vi "Check Incoming TP Timeouts.vi"(8 "error in":errorcluster, 11 "internal data":T1={"J1939 XNET Settings"={"XNET Database"="", "XNET Cluster"="", "CAN port"="", "Baud rate [Bd]"=0, "J1939 Network Address"=0, "Name"=0, "Termination"=0}, "j1939 queues"={"Processed Outgoing"=refnum, "Process Outgoing"=refnum, "stop notifier"=refnum, "error queue"=refnum, "active dtc"=refnum, "processed inc"=refnum}, "fgv references"={"BAM Buffer"=refnum, "CM Buffer"=refnum, "CM Gen"=refnum, "BAM Gen"=refnum, "Address Claims"=refnum, "RQST"=refnum, "scaling lut"=refnum, "data lut"=refnum, "cyclic scheduler"=refnum}, "frame in"="", "frame out"="", "timing"={"tb to j1939 queue timeout"=100, "j1939 to tb queue timeout"=100, "dtc loop period (ms)"=100, "CAN in loop period (ms)"=100, "process incoming queue timeout (ms)"=100, "Outgoing Write Decimation"=0, "process outgoing loop rate (ms)"=0, "periodic outgoing queue timeout (ms)"=10, "CAN out queue timeout (ms)"=100}}) -> (0 "error out":errorcluster)   [LabVIEW 2013, in "J1939.lvlib"]
uses:
  J1939.lvlib
  API Types/Internal Data.ctl
  API Types/XNET Settings.ctl
  API Types/Setup Information Cluster.ctl
  API Types/CAN Outgoing Message Cluster.ctl
  API Types/Convert DTCs Cluster.ctl
  <vilib>/xnet/xnet.llb/XNET Frame CAN.ctl
  <vilib>/xnet/xnet.llb/XNET Frame Type CAN.ctl
  TP List References.ctl
  BAM/BAM Buffer Connections List_Ref.ctl
  Connection Mode/Connection Mode Generation Connection Ref.ctl
  BAM/BAM Generation Connections List_Ref.ctl
  LUTs/J1939 Address Table Reference.ctl
  RQST/RQST Lookup Table Reference.ctl
  LUTs/J1939 Conversion Lookup Table Reference.ctl
  LUTs/J1939 Data Lookup Table Reference.ctl
  LUTs/Cyclic Frame Scheduler Lut Reference.ctl
  Configuration/TypeDefs/timing configuration.ctl
  TP Connections List State.ctl
  TP Buffer Check Timeout on Connections.vi
  Helpers/Buffer Connections List_Actions.vi
  Common Messages/J1939 Message TP.Conn Abort.vi
  Frame Conversion/Common Conversions.vi
  Frame Conversion/Convert J1939 ID to CAN Arb ID.vi
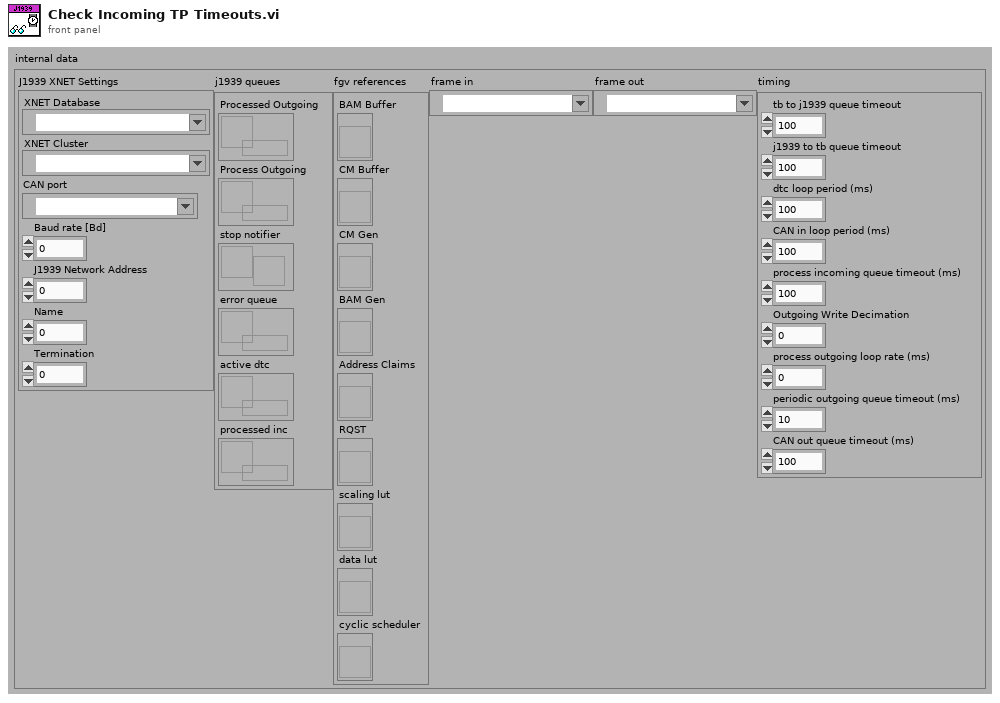
[diagram p1: front panel]
types:
  T1 = typedef "J1939.lvlib/Internal Data.ctl" = cluster{"J1939 XNET Settings":T2, "j1939 queues":T3, "fgv references":T4, "frame in":refnum<k21>, "frame out":refnum<k21>, "timing":T13}
  T2 = typedef "J1939.lvlib/XNET settings.ctl" = cluster{"XNET Database":refnum<k21>, "XNET Cluster":refnum<k21>, "CAN port":refnum<k21>, "Baud rate [Bd]":u32, "J1939 Network Address":u8, "Name":u64, "Termination":u32}
  T3 = typedef "J1939.lvlib/Setup Information Cluster.ctl" = cluster{"Processed Outgoing":refnum<queue>, "Process Outgoing":refnum<queue>, "stop notifier":refnum<notifier>, "error queue":refnum<queue>, "active dtc":refnum<queue>, "processed inc":refnum<queue>}
  T4 = typedef "J1939.lvlib/TP List References.ctl" = cluster{"BAM Buffer":T5, "CM Buffer":T5, "CM Gen":T6, "BAM Gen":T7, "Address Claims":T8, "RQST":T9, "scaling lut":T10, "data lut":T11, "cyclic scheduler":T12}
  T5 = typedef "J1939.lvlib/BAM Buffer Connections List_Ref.ctl" = refnum<vi>
  T6 = typedef "J1939.lvlib/Connection Mode Generation Connection Ref.ctl" = refnum<vi>
  T7 = typedef "J1939.lvlib/BAM Generation Connections List_Ref.ctl" = refnum<vi>
  T8 = typedef "J1939.lvlib/J1939 Address Table Reference.ctl" = refnum<vi>
  T9 = typedef "J1939.lvlib/RQST Lookup Table Reference.ctl" = refnum<vi>
  T10 = typedef "J1939.lvlib/J1939 Conversion Lookup Table Reference.ctl" = refnum<vi>
  T11 = typedef "J1939.lvlib/J1939 Data Lookup Table Reference.ctl" = refnum<vi>
  T12 = typedef "J1939.lvlib/cyclic frame scheduler lut reference.ctl" = refnum<vi>
  T13 = typedef "J1939.lvlib/timing configuration.ctl" = cluster{"tb to j1939 queue timeout":i32, "j1939 to tb queue timeout":i32, "dtc loop period (ms)":i32, "CAN in loop period (ms)":i32, "process incoming queue timeout (ms)":i32, "Outgoing Write Decimation":u32, "process outgoing loop rate (ms)":i32, "periodic outgoing queue timeout (ms)":i32, "CAN out queue timeout (ms)":i32}
  T14 = typedef "J1939.lvlib/TP Connections List State.ctl" = enum16{"Add", "Update", "Get", "Remove", "Initialize"}
  T15 = typedef "J1939.lvlib/TP Buffer Connection Cluster.ctl" = cluster{"Source Address":u8, "Destination Address":u8, "PGN":u32, "Arb ID":u32, "CAN Conversion Index":u32, "Total Expected Bytes":u16, "Total Expected Packets":u8, "Number of Packets Read":u8, "Start Time":u32, "Packets (U8)":u8[], "Timestamp":timestamp}
  T16 = typedef "J1939.lvlib/CAN Outgoing Message Cluster.ctl" = cluster{"Identifier":u32, "Data":u8[]}
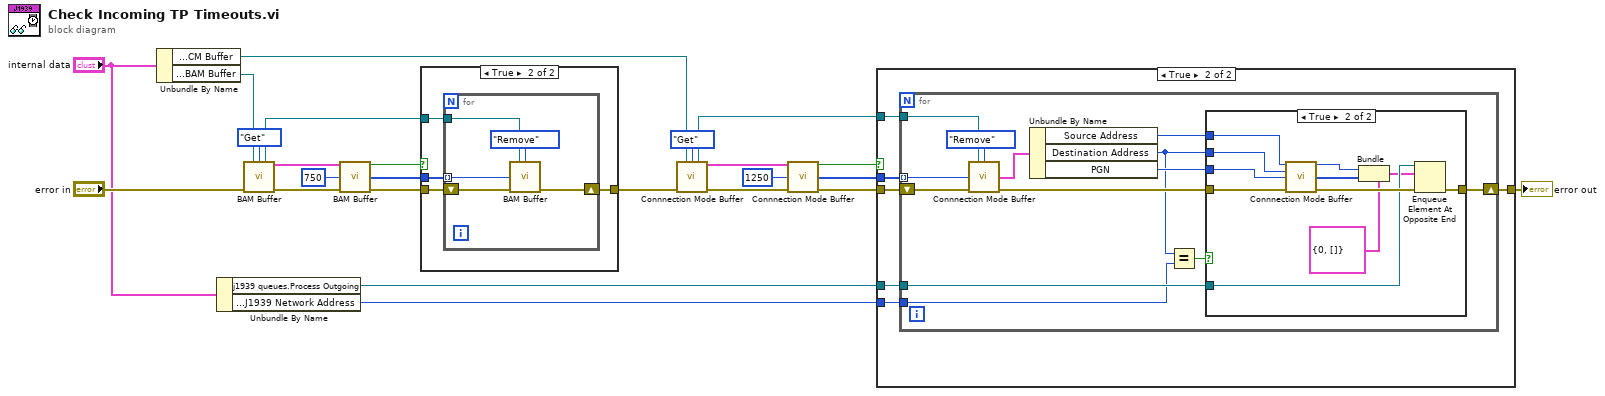
[diagram p0: block diagram]
diagram:
  n1 = Unbundle By Name("internal data") -> ("fgv references.CM Buffer"=w4:T5, "fgv references.BAM Buffer"=w5:T5)
  n2 = Unbundle By Name("internal data") -> ("j1939 queues.Process Outgoing"=w8:refnum<queue>, "J1939 XNET Settings.J1939 Network Address"=w2:u8)
  n3 = call-poly "BAM Buffer.vi"("ref in"=w5, "State"=TP_Connections_List_State."Get", "error in (no error)"="error in") -> ("ref out"=w6:T5, "Connections"=w11:T15[], "error out"=w12:errorcluster)  [unwired: 9 in, 1 out]
  n4 = call-poly "BAM Buffer.vi"("Connections"=w11, "Time Out"=u32 750, "error in (no error)"=w12) -> ("Timed Out Connections?"=w13:bool, "Index Array"=w14:i32[], "error out"=w15:errorcluster)  [unwired: 10 out]
  n5 = case shown="True" w13 {
    tunnel: w14 -> [_ w29]
    tunnel: w15 -> [w25 w28]
    tunnel: [w25 w27] -> w17
    tunnel: w6 -> [_ w26]
    frame False {
    }
    frame True {
      n6 = for {
        tunnel: w29 -> [w33] mode=indexing
        shift-right: [w31] -> w27
        shift-left: w28 -> [w32]
        tunnel: w26 -> [w30]
        n7 = call-poly "BAM Buffer.vi"("ref in"=w30, "State"=TP_Connections_List_State."Remove", "index"=w33, "error in (no error)"=w32) -> ("error out"=w31:errorcluster)  [unwired: 8 in, 3 out]
      }
    }
  }
  n8 = call-poly "Connnection Mode Buffer.vi"("ref in"=w4, "State"=TP_Connections_List_State."Get", "error in (no error)"=w17) -> ("ref out"=w3:T5, "Connections"=w20:T15[], "error out"=w16:errorcluster)  [unwired: 2 in, 8 out]
  n9 = call-poly "Connnection Mode Buffer.vi"("Connections"=w20, "Time Out"=u32 1250, "error in (no error)"=w16) -> ("Timed Out Connections?"=w23:bool, "Index Array"=w22:i32[], "error out"=w21:errorcluster)  [unwired: 10 out]
  n10 = case shown="True" w23 {
    tunnel: w22 -> [_ w41]
    tunnel: w21 -> [w35 w40]
    tunnel: [w35 w39] -> w24
    tunnel: w8 -> [_ w38]
    tunnel: w3 -> [_ w37]
    tunnel: w2 -> [_ w36]
    frame False {
    }
    frame True {
      n11 = for {
        tunnel: w41 -> [w53] mode=indexing
        shift-right: [w47] -> w39
        shift-left: w40 -> [w54]
        tunnel: w38 -> [w46]
        tunnel: w37 -> [w45]
        tunnel: w36 -> [w44]
        n12 = call-poly "Connnection Mode Buffer.vi"("ref in"=w45, "State"=TP_Connections_List_State."Remove", "index"=w53, "error in (no error)"=w54) -> ("Connection Cluster Out"=w50:T15, "error out"=w51:errorcluster)  [unwired: 1 in, 9 out]
        n13 = Unbundle By Name(w50) -> ("Source Address"=w49:u8, "Destination Address"=w43:u8, "PGN"=w48:u32)
        n14 = Equal?(x=w43, y=w44) -> (x = y?=w42:bool)
        n15 = case shown="True" w42 {
          tunnel: w51 -> [w55 w66]
          tunnel: w49 -> [_ w65]
          tunnel: w43 -> [_ w64]
          tunnel: w48 -> [_ w63]
          tunnel: [w55 w61] -> w47
          tunnel: w46 -> [_ w60]
          frame False {
          }
          frame True {
            n16 = call-poly "Connnection Mode Buffer.vi"("Destination Address"=w65, "Source Address"=w64, "PGN"=w63, "error in (no error)"=w66) -> ("Arb ID"=w59:u32, "Data"=w58:u8[], "error out"=w62:errorcluster)  [unwired: 9 out]
            n17 = Bundle(cluster=T16 {"Identifier"=0, "Data"=[]} ("Data to Send"), "Identifier"=w59, "Data"=w58) -> (w56:T16)
            n18 = Enqueue Element At Opposite End(queue=w60, element=w56, error in (no error)=w62) -> (error out=w61:errorcluster)  [unwired: 3 out]
          }
        }
      }
    }
  }
  "error out" <- w24
